vi "TP.vi"(8 "Cluster in":refnum<vi>, 10 "Time":i32, 11 "Trigger":bool) -> (2 "ET 4":i32, 3 "Q 4":bool)   [LabVIEW 2020]
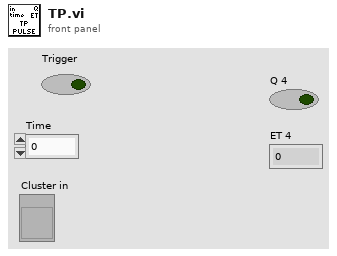
[diagram p1: front panel]
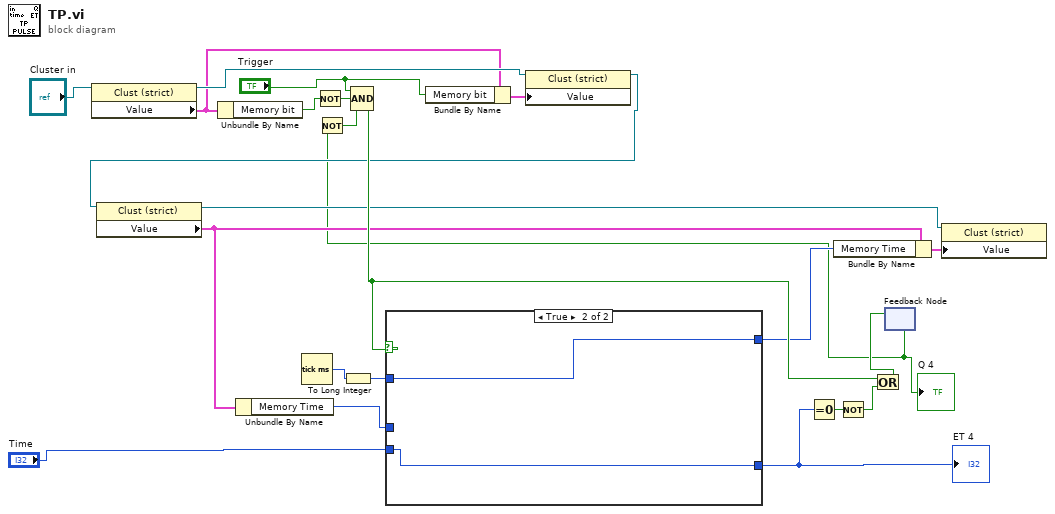
[diagram p0: block diagram]
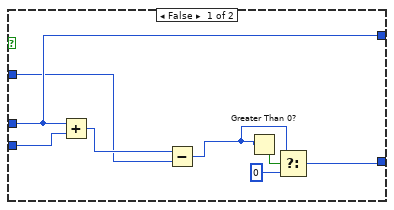
[diagram p2: hidden frame]
diagram:
  n1 = property class="Clust (strict)"(reference="Cluster in") -> (reference out=w9:refnum<vi>, "Value"=w8:cluster{"Memory bit":bool, "Memory Time":i32})  [unwired: 1 in, 1 out]
  n2 = Unbundle By Name(w8) -> ("Memory bit"=w6:bool)
  n3 = Tick Count (ms)() -> (millisecond timer value=w13:u32)
  n4 = Not(x=w6) -> (.not. x?=w20:bool)
  n5 = To Long Integer(number=w13) -> (32bit integer=w12:i32)
  n6 = Bundle By Name(cluster=w8, "Memory bit"="Trigger") -> (w7:cluster{"Memory bit":bool, "Memory Time":i32})
  n7 = property class="Clust (strict)"(reference=w9, "Value"=w7) -> (reference out=w19:refnum<vi>)  [unwired: 1 in, 1 out]
  n8 = property class="Clust (strict)"(reference=w19) -> (reference out=w18:refnum<vi>, "Value"=w16:cluster{"Memory bit":bool, "Memory Time":i32})  [unwired: 1 in, 1 out]
  n9 = Unbundle By Name(w16) -> ("Memory Time"=w14:i32)
  n10 = feedback #1() -> (w3:bool)  [unwired: 1 in]
  "Q 4" <- w3
  n11 = Not(x=w3) -> (.not. x?=w21:bool)
  n12 = Compound Arithmetic op=AND("Trigger", w20, w21) -> (w22:bool)
  n13 = case shown="True" w22 {
    tunnel: w12 -> [w25 w33]
    tunnel: [w26 w33] -> w17
    tunnel: w14 -> [w26 _]
    tunnel: "Time" -> [w27 w32]
    tunnel: [w24 w32] -> w2
    frame False {
      n14 = Add(x=w26, y=w27) -> (x+y=w31:i32)
      n15 = Subtract(x=w31, y=w25) -> (x-y=w29:i32)
      n16 = Greater Than 0?(x=w29) -> (x > 0?=w30:bool)
      n17 = Select(t=w29, s=w30, f=0) -> (s? t:f=w24:i32)
    }
    frame True {
    }
  }
  "ET 4" <- w2
  n18 = Equal To 0?(x=w2) -> (x = 0?=w11:bool)
  n19 = Bundle By Name(cluster=w16, "Memory Time"=w17) -> (w15:cluster{"Memory bit":bool, "Memory Time":i32})
  n20 = Not(x=w11) -> (.not. x?=w10:bool)
  n21 = Or(x=w22, y=w10) -> (x .or. y?=w23:bool)
  n22 = feedback-in #1(w23) -> ()
  n23 = property class="Clust (strict)"(reference=w18, "Value"=w15) -> ()  [unwired: 1 in, 2 out]
